vi "Grave Left Cell String.vi"(8 "Error In":errorcluster, 10 "Bookmark ID":u32, 11 "VI Path":path) -> (0 "Error Out":errorcluster, 3 "Text":string)   [LabVIEW 2017, in "Graveyard.lvlib"]
doc: "Gets the state name of the grave. If the Spirit frame is enabled, then the name is \"Spirit\". If the Corpse frame is enabled, then the name is \"Zombie\".\n\nThe Diagram Disable Structure cannot be obtained its label. The owning object of the label is the block diagram, not the Diagram Disable Structure that is attached to it. This means that all of the Diagram Disable structures in a VI must be searched by their label's UIDs to find the Diagram Disable Structure and determine its state."
uses:
  Graveyard.lvlib
  <vilib>/Utility/traverseref.llb/TRef TravTarget.ctl
  Eulogy/Public/Grave States.ctl
  <vilib>/Utility/traverseref.llb/VI Scripting - Traverse.lvlib
  Eulogy/Eulogy.lvlib
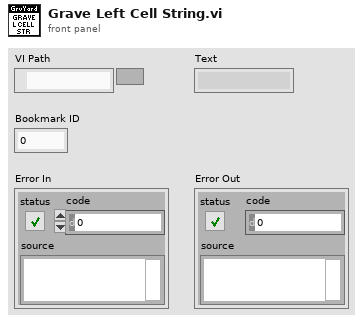
[diagram p1: front panel]
types:
  T1 = typedef "TRef TravTarget.ctl" = enum16{"FP", "BD", "Other"}
  T2 = typedef "Eulogy.lvlib/Grave States.ctl" = enum16{"Spirit", "Zombie"}
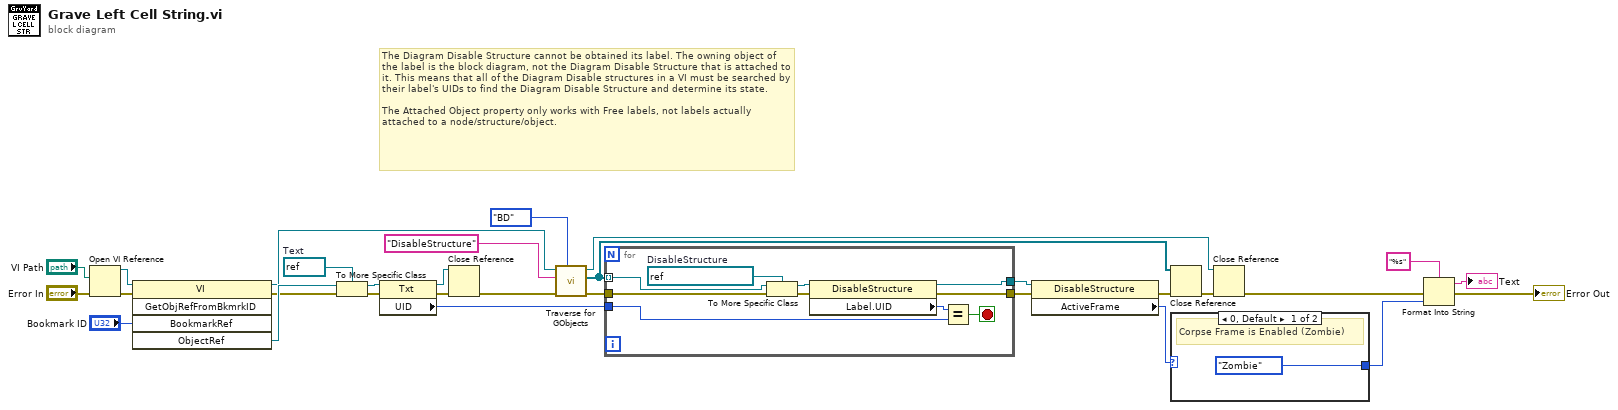
[diagram p0: block diagram]
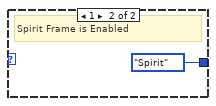
[diagram p2: hidden frame]
diagram:
  w19 = refnum<vi> refnum  # Text
  # "The Diagram Disable Structure cannot be obtained its label. The owning object of the label is the block diagram, not the Diagram Disable Structure that is attached to it. This means that all of the Diagram Disable structures in a VI must be searched by their label's UIDs to find the Diagram Disable Structure and determine its state.\n\nThe Attached Object property only works with Free labels, not labels actually attached to a node/structure/object."
  n1 = Open VI Reference(vi path="VI Path", error in (no error)="Error In") -> (vi reference=w11:refnum<vi>, error out=w12:errorcluster)  [unwired: 4 in]
  n2 = invoke class="VI" method="GetObjRefFromBkmrkID"(reference=w11, error in=w12, "BookmarkRef"="Bookmark ID") -> (reference out=w7:refnum<vi>, error out=w18:errorcluster, "ObjectRef"=w21:refnum<vi>)  [unwired: 2 in, 2 out]
  n3 = To More Specific Class(target class=w19, reference=w21, error in=w18) -> (specific class reference=w22:refnum<vi>, error out=w20:errorcluster)
  n4 = property class="Txt"(reference=w22, error in=w20) -> (reference out=w5:refnum<vi>, error out=w9:errorcluster, "UID"=w25:i32)
  n5 = Close Reference(reference=w5, error in (no error)=w9) -> (error out=w6:errorcluster)
  n6 = call <vilib>:"Traverse for GObjects.vi"("Traverse Target"=TRef_TravTarget."BD", "error in (no error)"=w6, "Class Name"="DisableStructure", "VI Refnum"=w7) -> ("error out"=w8:errorcluster, "References"=w30:refnum<vi>[], "dup VI Refnum"=w10:refnum<vi>)  [unwired: 4 in, 1 out]
  n7 = for {
    tunnel: w30 -> [w40] mode=indexing
    tunnel: w25 -> [w33]
    tunnel: w8 -> [w38]
    tunnel: [w36] -> w26
    tunnel: [w32] -> w28
    stop <- w31 stop-if-true
    w39 = refnum<vi> refnum  # DisableStructure
    n8 = To More Specific Class(target class=w39, reference=w40, error in=w38) -> (specific class reference=w35:refnum<vi>, error out=w37:errorcluster)
    n9 = property class="DisableStructure"(reference=w35, error in=w37) -> (reference out=w32:refnum<vi>, error out=w36:errorcluster, "Label.UID"=w34:i32)
    n10 = Equal?(x=w34, y=w33) -> (x = y?=w31:bool)
  }
  n11 = property class="DisableStructure"(reference=w28, error in=w26) -> (error out=w27:errorcluster, "ActiveFrame"=w29:i16)  [unwired: 1 out]
  n12 = Close Reference(reference=w30, error in (no error)=w27) -> (error out=w16:errorcluster)
  n13 = case shown="0, Default" w29 {
    tunnel: [Grave_States."Zombie" ("Grave States") Grave_States."Spirit" ("Grave States")] -> w3
    frame 0, Default {
      # "Corpse Frame is Enabled (Zombie)"
    }
    frame 1 {
      # "Spirit Frame is Enabled"
    }
  }
  n14 = Close Reference(reference=w10, error in (no error)=w16) -> (error out=w17:errorcluster)
  n15 = Format Into String(format string="%s", error in=w17, w3) -> (resulting string=→"Text":string, error out=→"Error Out":errorcluster)  [unwired: 1 in]
